vi "GetPosition.vi"(10 "RPM Update Data":T1, 11 "Time":timestamp) -> (1 "Arduino Timeout":bool, 2 "Speed (RPM)":dbl, 3 "Position (deg)":dbl)   [LabVIEW 2014]
uses:
  RPMUpdateData.ctl
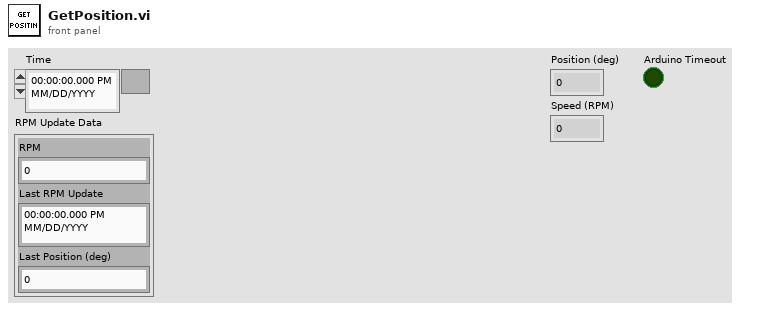
[diagram p1: front panel]
types:
  T1 = typedef "RPMUpdateData.ctl" = cluster{"RPM":dbl, "Last RPM Update":timestamp, "Last Position (deg)":dbl}
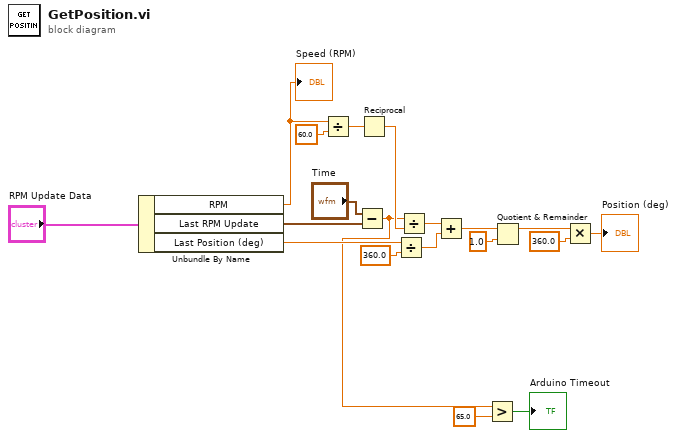
[diagram p0: block diagram]
diagram:
  n1 = Unbundle By Name("RPM Update Data") -> ("RPM"=w19:dbl, "Last RPM Update"=w16:timestamp, "Last Position (deg)"=w6:dbl)
  "Speed (RPM)" <- w19
  n2 = Divide(x=w19, y=60.0) -> (x/y=w17:dbl)
  n3 = Subtract(x="Time", y=w16) -> (x-y=w3:dbl)
  n4 = Reciprocal(x=w17) -> (1/x=w15:dbl)
  n5 = Divide(x=w6, y=360.0) -> (x/y=w12:dbl)
  n6 = Divide(x=w3, y=w15) -> (x/y=w13:dbl)
  n7 = Add(x=w13, y=w12) -> (x+y=w11:dbl)
  n8 = Greater?(x=w3, y=65.0) -> (0:→"Arduino Timeout":bool)
  n9 = Quotient & Remainder(x=w11, y=1.0) -> (x-y*floor(x/y)=w9:dbl)  [unwired: 1 out]
  n10 = Multiply(x=w9, y=360.0) -> (x*y=→"Position (deg)":dbl)
